vi "Zero.vi"(0 "RS NRPx Power Meter in":refnum<class "Power Meter.lvclass">, 11 "error in":errorcluster) -> (4 "RS NRPx Power Meter out":refnum<class "Power Meter.lvclass">, 15 "error out":errorcluster)   [LabVIEW 2023, in "RS NRPx Power Meter.lvlib" / "Power Meter.lvclass"]
uses:
  Power Meter.lvclass
  Power Meter.lvclass/Power Meter.ctl
  Properties/Read Resource Name.vi
  <instrlib>/Rohde&Schwarz Power Meter/Rohde&Schwarz Power Meter.lvlib
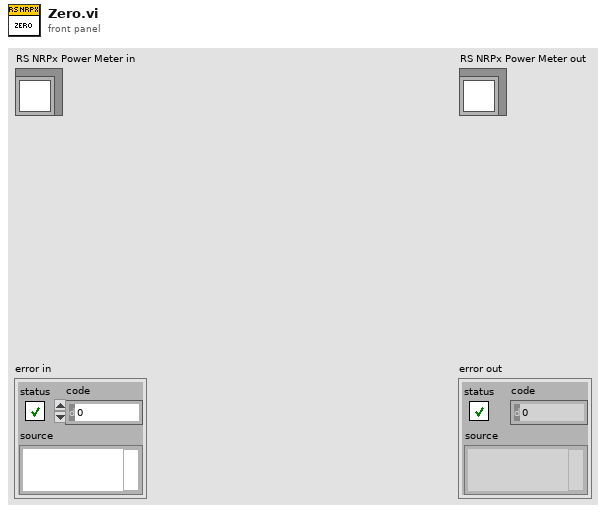
[diagram p1: front panel]
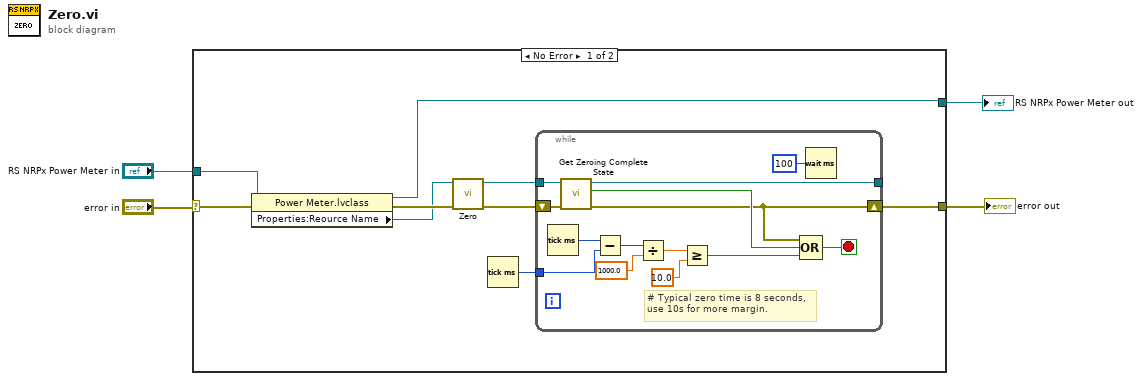
[diagram p0: block diagram]
diagram:
  n1 = case shown="No Error" "error in" {
    selector: "error in" -> [w13 w29]
    tunnel: [w6 w29] -> w1
    tunnel: "RS NRPx Power Meter in" -> [w12 w28]
    tunnel: [w11 w28] -> w2
    frame No Error {
      n2 = property class="Power Meter.lvclass"(reference=w12, error in=w13) -> (reference out=w11:refnum<class "Power Meter.lvclass">, error out=w10:errorcluster, "Properties:Reource Name"=w5:refnum<visa-resource-name>)
      n3 = call <instrlib>:"Zero.vi"("error in (no error)"=w10, "VISA resource name"=w5) -> ("error out"=w9:errorcluster, "VISA resource name out"=w8:refnum<visa-resource-name>)  [unwired: 8 in]
      n4 = Tick Count (ms)() -> (millisecond timer value=w7:u32)
      n5 = while {
        tunnel: w8 -> [w21]
        shift-right: [w14] -> w6
        shift-left: w9 -> [w20]
        tunnel: w7 -> [w26]
        tunnel: [w18] -> _
        stop <- w22 stop-if-true
        # "# Typical zero time is 8 seconds,\nuse 10s for more margin."
        n6 = Tick Count (ms)() -> (millisecond timer value=w27:u32)
        n7 = call <instrlib>:"Get Zeroing Complete State.vi"("error in (no error)"=w20, "VISA resource name"=w21) -> ("error out"=w14:errorcluster, "Zeroing Complete"=w19:bool, "VISA resource name out"=w18:refnum<visa-resource-name>)  [unwired: 7 in]
        n8 = Subtract(x=w27, y=w26) -> (x-y=w25:u32)
        n9 = Divide(x=w25, y=1000.0 ("timer")) -> (x/y=w17:dbl)
        n10 = Greater Or Equal?(x=w17, y=10.0) -> (x >= y?=w23:bool)
        n11 = Compound Arithmetic op=OR(w14, w19, w23) -> (w22:bool)
        n12 = Wait (ms)(milliseconds to wait=u32 100) -> ()  [unwired: 1 out]
      }
    }
    frame Error {
    }
  }
  "error out" <- w1
  "RS NRPx Power Meter out" <- w2
